vi "Check If Error Exists.vi"(8 "error in":errorcluster, 10 "error key":string, 11 "section ref in":T1 format="%.0x") -> (0 "error out":errorcluster, 2 "error exists?":bool, 3 "section ref out":T1 format="%.0x")   [LabVIEW 2023, in "Ballard MIL-STD-1553 Scripting.lvlib"]
uses:
  Ballard MIL-STD-1553 Scripting.lvlib
  NationalInstruments.VeriStand.SystemDefinitionAPI
  NationalInstruments.VeriStand.SystemStorage
  <vilib>/NI VeriStand/Custom Device API/Custom Device Item Ref.ctl
  <vilib>/NI VeriStand/Custom Device API/Custom Device API.lvlib
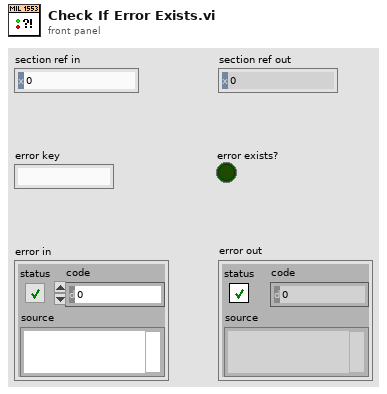
[diagram p1: front panel]
types:
  T1 = typedef "Custom Device API.lvlib/Custom Device Item Ref.ctl" = u64
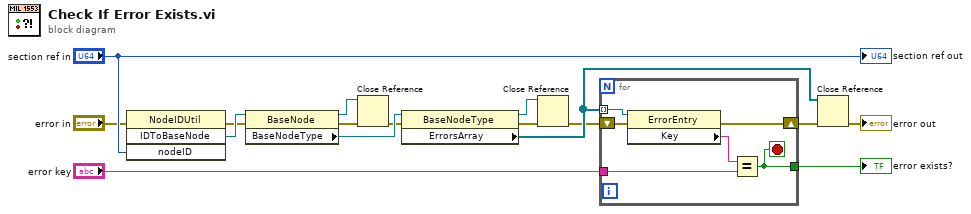
[diagram p0: block diagram]
diagram:
  n1 = invoke on="Invoke Node" class="NodeIDUtil" method="IDToBaseNode"(error in="error in", "nodeID"="section ref in") -> (error out=w11:errorcluster, "IDToBaseNode"=w16:refnum<k24>)  [unwired: 2 in, 2 out]
  n2 = property on="Property Node" class="BaseNode"(reference=w16, error in=w11) -> (reference out=w7:refnum<k24>, error out=w12:errorcluster, "BaseNodeType"=w15:refnum<k24>)
  n3 = Close Reference(reference=w7, error in (no error)=w12) -> (error out=w8:errorcluster)
  n4 = property on="Property Node" class="BaseNodeType"(reference=w15, error in=w8) -> (reference out=w5:refnum<k24>, error out=w13:errorcluster, "ErrorsArray"=w10:refnum<k24>[])
  n5 = Close Reference(reference=w5, error in (no error)=w13) -> (error out=w6:errorcluster)
  n6 = for {
    tunnel: w10 -> [w22] mode=indexing
    shift-right: [w21] -> w14
    shift-left: w6 -> [w20]
    tunnel: "error key" -> [w18]
    tunnel: [w17] -> w9
    stop <- w17 stop-if-true
    n7 = property on="Property Node" class="ErrorEntry"(reference=w22, error in=w20) -> (error out=w21:errorcluster, "Key"=w19:string)  [unwired: 1 out]
    n8 = Equal?(x=w19, y=w18) -> (x = y?=w17:bool)
  }
  "error exists?" <- w9
  n9 = Close Reference(reference=w10, error in (no error)=w14) -> (error out=→"error out":errorcluster)
  "section ref out" <- "section ref in"
